vi "Check_Angles.vi"(10 "Joint positions (rad)":dbl[](array[numeric])) -> (2 "Adjusted joint positions (rad)":dbl[](array[numeric]))   [LabVIEW 2015]
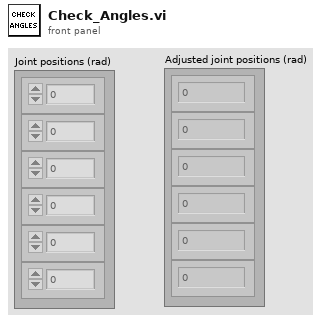
[diagram p1: front panel]
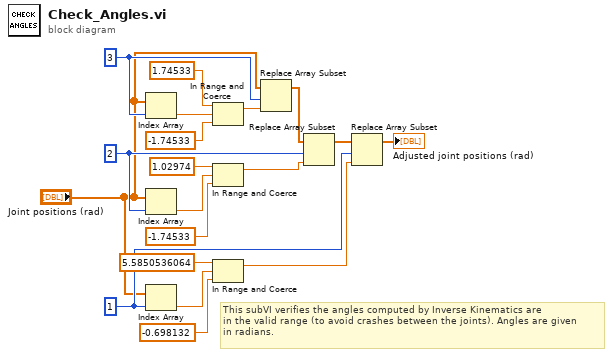
[diagram p0: block diagram]
diagram:
  w6 = 1 ("index")
  w11 = 2 ("index")
  w16 = 3 ("index")
  # "This subVI verifies the angles computed by Inverse Kinematics are\nin the valid range (to avoid crashes between the joints). Angles are given\nin radians."
  n1 = Index Array(array="Joint positions (rad)", index=w16) -> (element=w19:dbl)
  n2 = Index Array(array="Joint positions (rad)", index=w11) -> (element=w14:dbl)
  n3 = Index Array(array="Joint positions (rad)", index=w6) -> (element=w4:dbl)
  n4 = In Range and Coerce(upper limit=1.74533, x=w19, lower limit=-1.74533) -> (coerced(x)=w15:dbl)  [unwired: 1 out]
  n5 = In Range and Coerce(upper limit=1.02974, x=w14, lower limit=-1.74533) -> (coerced(x)=w10:dbl)  [unwired: 1 out]
  n6 = In Range and Coerce(upper limit=5.5850536064, x=w4, lower limit=-0.698132) -> (coerced(x)=w5:dbl)  [unwired: 1 out]
  n7 = Replace Array Subset(array="Joint positions (rad)", new element=w15, index=w16) -> (w9:dbl[])
  n8 = Replace Array Subset(array=w9, new element=w10, index=w11) -> (w8:dbl[])
  n9 = Replace Array Subset(array=w8, new element=w5, index=w6) -> (→"Adjusted joint positions (rad)":dbl[])
